vi "Close Session.vi"(8 "error in (no error)":errorcluster, 11 "MB TCP session":refnum<class "MB_Master_TCP.lvclass">) -> (0 "error out":errorcluster)   [LabVIEW 2016, in "MB Master.lvlib" / "MB_Master_TCP.lvclass"]
doc: "Close the Modbus session. This will release the mutex and close the TCP connection."
uses:
  MB_Master_TCP.lvclass
  MB_Master_TCP.lvclass/MB_Master_TCP.ctl
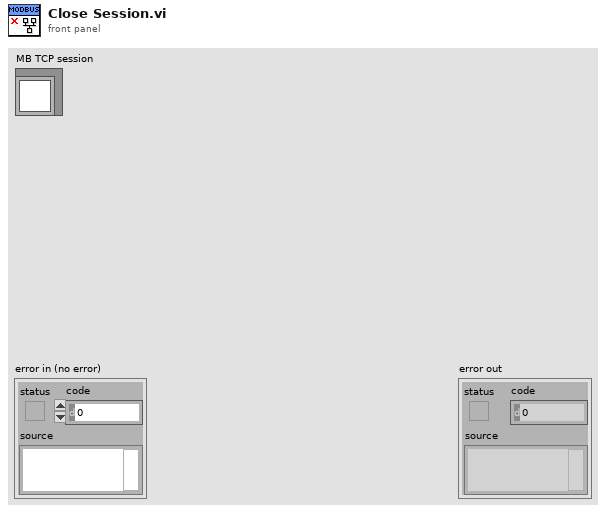
[diagram p1: front panel]
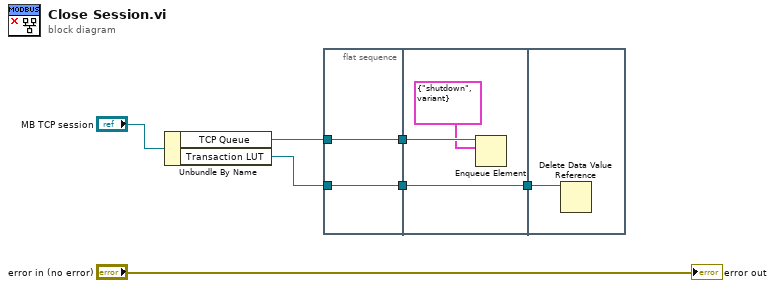
[diagram p0: block diagram]
diagram:
  n1 = Unbundle By Name("MB TCP session") -> ("TCP Queue"=w6:refnum<queue>, "Transaction LUT"=w2:refnum<data-value>)
  n2 = flat-sequence {
    tunnel: w6 -> [w9]
    tunnel: [w9] -> w4
    tunnel: [w8] -> w3
    tunnel: w2 -> [w8]
    tunnel: w4 -> [w12]
    tunnel: w3 -> [w10]
    tunnel: [w10] -> w1
    tunnel: w1 -> [w13]
    frame #0 {
    }
    frame #1 {
      n3 = Enqueue Element(queue=w12, element=cluster{"cmd":string, "data":variant} {"cmd"="shutdown", "data"=variant}) -> ()  [unwired: 2 in, 3 out]
    }
    frame #2 {
      n4 = Delete Data Value Reference(data value reference=w13) -> ()  [unwired: 1 in, 2 out]
    }
  }
  "error out" <- "error in (no error)"
